vi "ASI_zero.vi"(2 "error in (no error)":errorcluster, 3 "VISA resource name":refnum<visa-resource-name>="COM7") -> (0 "error out":errorcluster, 1 "VISA resource name out":refnum<visa-resource-name>)   [LabVIEW 2015]
uses:
  <vilib>/Instr/_visa.llb/VISA Flush IO Buffer Mask.ctl
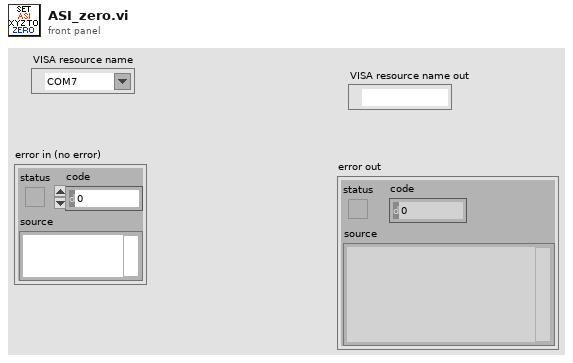
[diagram p1: front panel]
types:
  T1 = typedef "VISA Flush IO Buffer Mask.ctl" = u16
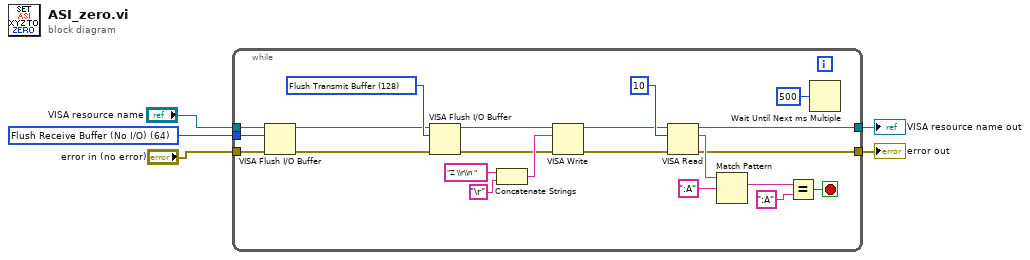
[diagram p0: block diagram]
diagram:
  w4 = T1 64 items=["Flush Receive Buffer"=16, "Write Transmit Buffer to Device"=32, "Flush Receive Buffer (No I/O)"=64, "Flush Transmit Buffer"=128] ("Mask")
  n1 = while {
    tunnel: "error in (no error)" -> [w25]
    tunnel: w4 -> [w19]
    tunnel: "VISA resource name" -> [w18]
    tunnel: [w11] -> w2
    tunnel: [w7] -> w1
    stop <- w10 stop-if-true
    w22 = T1 128 items=["Flush Receive Buffer"=16, "Write Transmit Buffer to Device"=32, "Flush Receive Buffer (No I/O)"=64, "Flush Transmit Buffer"=128] ("Mask")
    n2 = VISA Flush I/O Buffer(VISA resource name=w18, mask (16)=w19, error in (no error)=w25) -> (VISA resource name out=w21:refnum<visa-resource-name>, error out=w20:errorcluster)
    n3 = VISA Flush I/O Buffer(VISA resource name=w21, mask (16)=w22, error in (no error)=w20) -> (VISA resource name out=w24:refnum<visa-resource-name>, error out=w23:errorcluster)
    n4 = Concatenate Strings("Z \\r\\n " ("format string"), "\r") -> (w26:string)
    n5 = VISA Write(VISA resource name=w24, write buffer=w26, error in (no error)=w23) -> (VISA resource name out=w8:refnum<visa-resource-name>, error out=w12:errorcluster)  [unwired: 1 out]
    n6 = VISA Read(VISA resource name=w8, byte count=u32 10, error in (no error)=w12) -> (VISA resource name out=w7:refnum<visa-resource-name>, read buffer=w15:string, error out=w11:errorcluster)  [unwired: 1 out]
    n7 = Match Pattern(string=w15, regular expression=":A" ("y")) -> (match substring=w16:string)  [unwired: 1 in, 3 out]
    n8 = Equal?(x=w16, y=":A") -> (x = y?=w10:bool)
    n9 = Wait Until Next ms Multiple(millisecond multiple=u32 500) -> ()  [unwired: 1 out]
  }
  "error out" <- w2
  "VISA resource name out" <- w1
